vi "_Data Manager.vi"(5 "Error IN":errorcluster, 8 "Action":T1) -> (14 "Table":string[][](table), 19 "Error OUT":errorcluster)   [LabVIEW 2011]
uses:
  Controls/Data Manager Action.ctl
  Driver/Serial RS485/Controls/Serial_Action_Enum.ctl
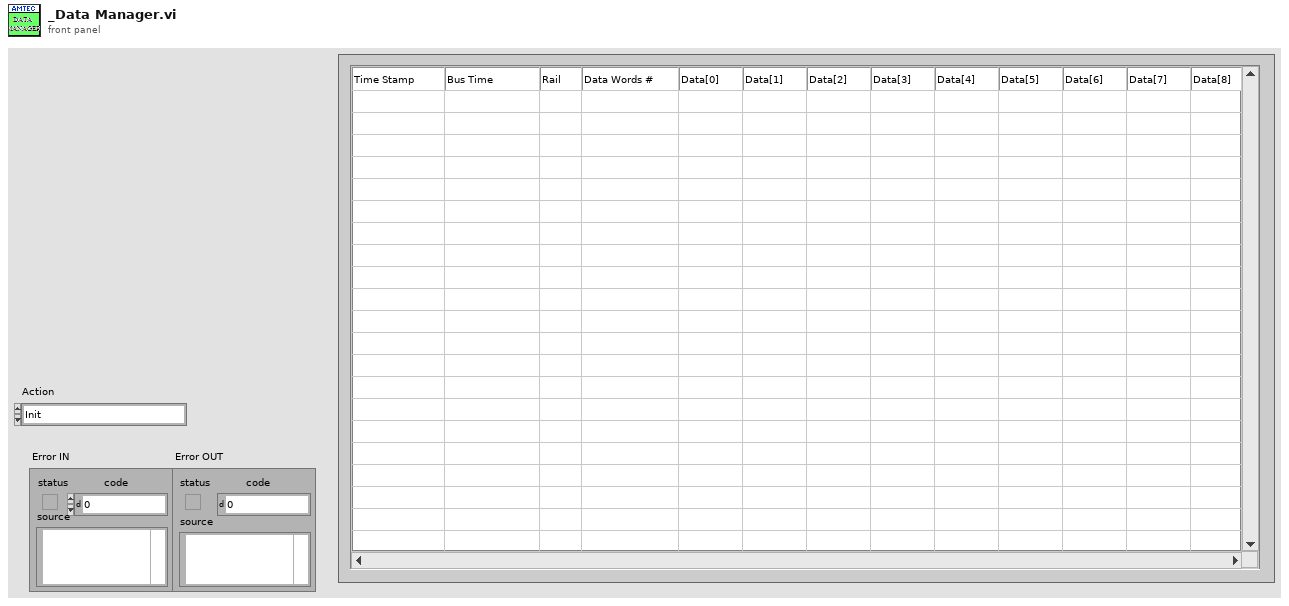
[diagram p1: front panel]
types:
  T1 = typedef "Data Manager Action.ctl" = enum16{"Init", "Status", "Get Data", "Get Log File Path", "Write Header", "Log Data", "Clear Table Data"}
  T2 = typedef "Serial_Action_Enum.ctl" = enum16{"Init", "Status", "Close", "Read All Chan", "Set Read Start Bit", "Clear Read Start Bit", "Read Beat", "Set RS485 Settings", "Close Ref"}
  T3 = typedef "Serial Data Cluster.ctl" = cluster{"String_Chan_1":string, "String_Chan_2":string, "String_Chan_3":string, "String_Chan_4":string, "#of Element Read Chan _1":i32, "#of Element Read Chan _2":i32, "#of Element Read Chan _3":i32, "#of Element Read Chan _4":i32, "Chan_1":timestamp, "Chan_2":timestamp, "Chan_3":timestamp, "Chan_4":timestamp}
  T4 = cluster{"Main Panel Path":path, "Config Directory":path, "Log Directory":path}
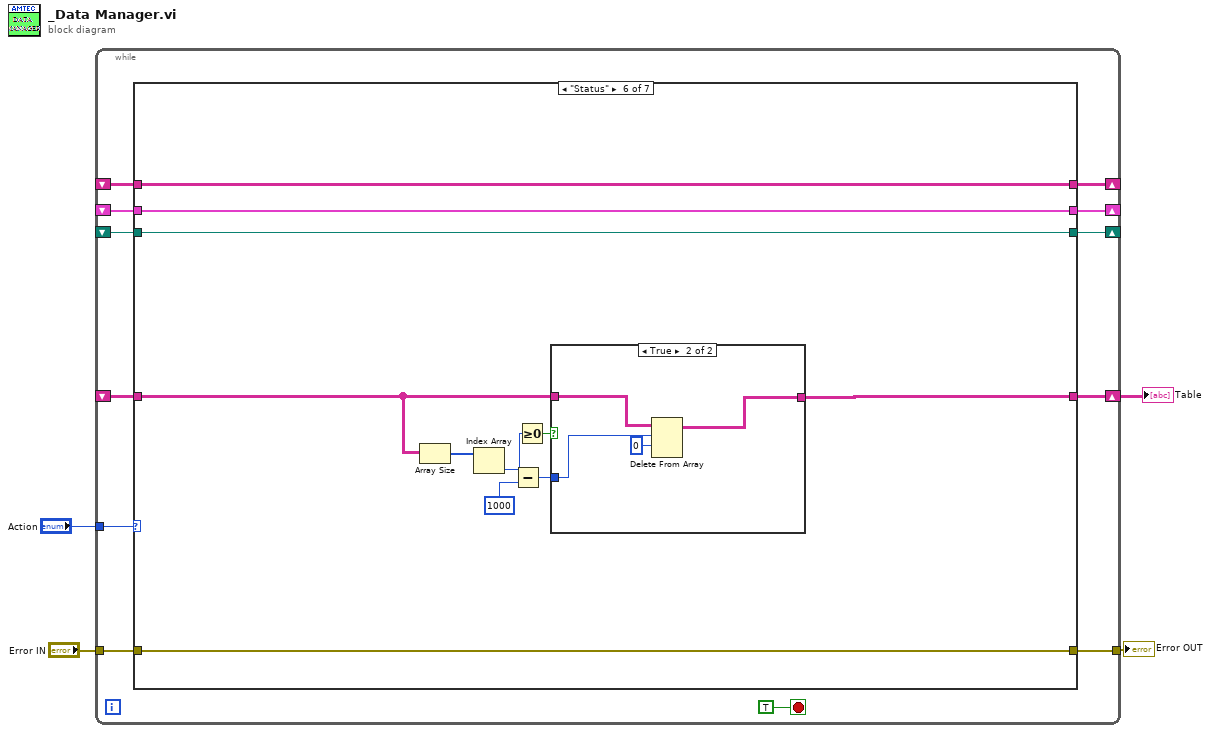
[diagram p0: block diagram]
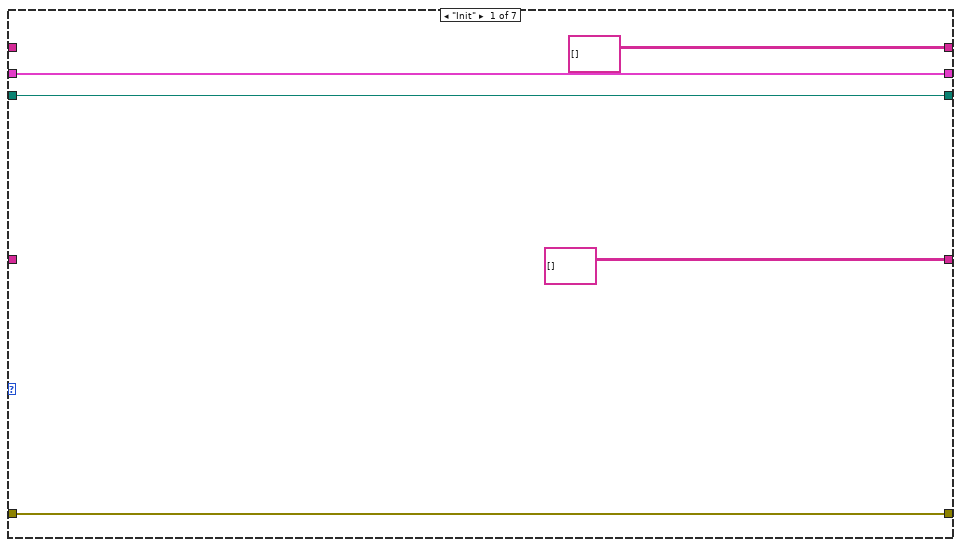
[diagram p2: hidden frame]
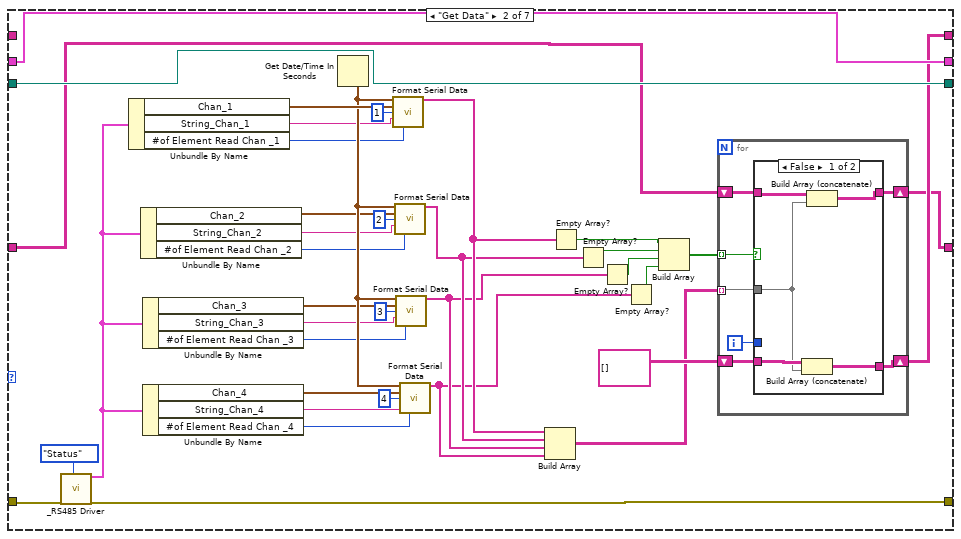
[diagram p3: hidden frame]
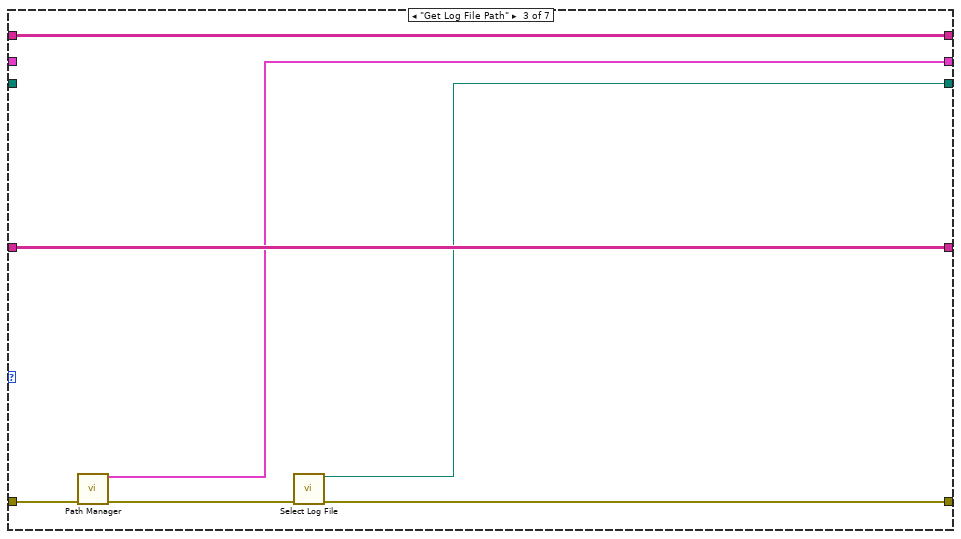
[diagram p5: hidden frame]
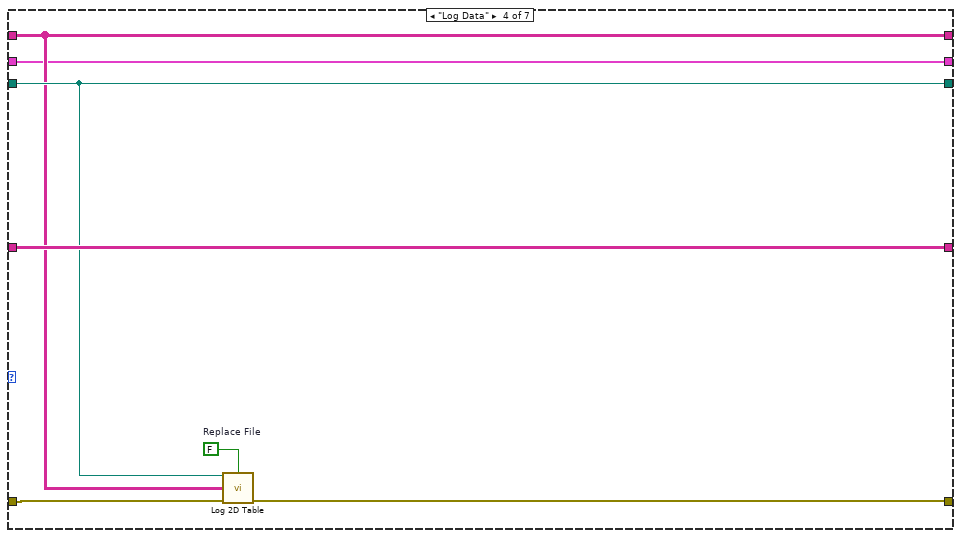
[diagram p6: hidden frame]
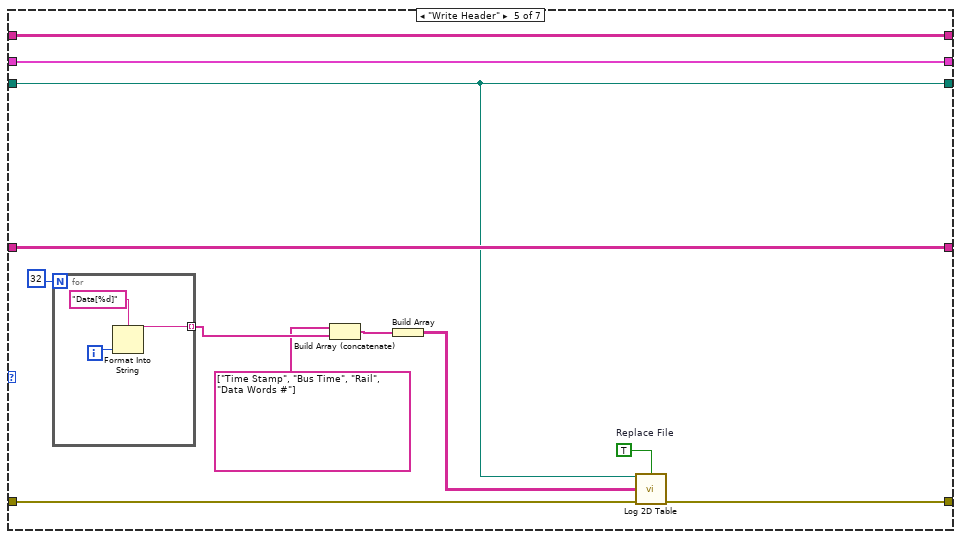
[diagram p7: hidden frame]
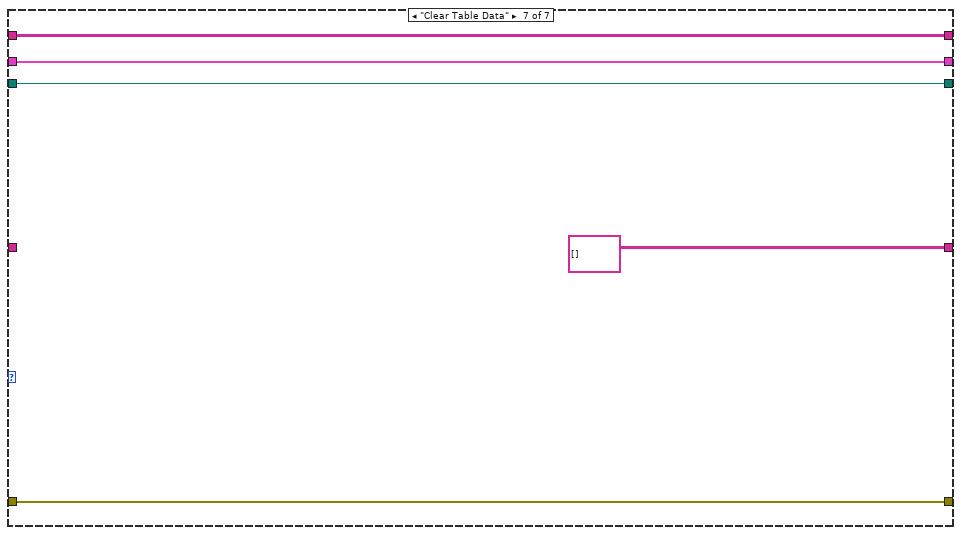
[diagram p9: hidden frame]
diagram:
  n1 = while {
    tunnel: "Action" -> [w15]
    tunnel: "Error IN" -> [w14]
    tunnel: [w13] -> w3
    shift-right: [w12] -> w1
    shift-left: _ -> [w11]
    shift-right: [w10] -> _
    shift-left: _ -> [w9]
    shift-right: [w8] -> _
    shift-left: _ -> [w7]
    shift-right: [w6] -> _
    shift-left: _ -> [w5]
    stop <- TRUE stop-if-true
    n2 = case shown="\"Status\"" w15 {
      tunnel: w14 -> [w21 w58 w77 w85 w93 w112 w122]
      tunnel: [w21 w57 w73 w82 w91 w112 w122] -> w13
      tunnel: [string[][] [] ("Results Table") w22 w79 w86 w98 w104 string[][] [] ("Results Table")] -> w12
      tunnel: w11 -> [_ w31 w79 w86 w98 w105 _]
      tunnel: [string[][] [] w23 w78 w83 w97 w111 w121] -> w10
      tunnel: w9 -> [_ _ w78 w83 w97 w111 w121]
      tunnel: [w18 w37 w76 w81 w88 w110 w120] -> w8
      tunnel: w7 -> [w18 w37 _ w81 w88 w110 w120]
      tunnel: [w17 w36 w74 w84 w92 w109 w119] -> w6
      tunnel: w5 -> [w17 w36 _ w84 w92 w109 w119]
      frame "Init" {
      }
      frame "Get Data" {
        n3 = call "_RS485 Driver.vi"("Error IN"=w58, "Action"=Serial_Action_Enum."Status") -> ("Serial Data Out"=w46:T3, "Error OUT"=w57:errorcluster)  [unwired: 15 in, 1 out]
        n4 = Unbundle By Name(w46) -> ("Chan_1"=w55:timestamp, "String_Chan_1"=w38:string, "#of Element Read Chan _1"=w45:i32)
        n5 = Unbundle By Name(w46) -> ("Chan_2"=w51:timestamp, "String_Chan_2"=w39:string, "#of Element Read Chan _2"=w44:i32)
        n6 = Unbundle By Name(w46) -> ("Chan_3"=w52:timestamp, "String_Chan_3"=w40:string, "#of Element Read Chan _3"=w43:i32)
        n7 = Unbundle By Name(w46) -> ("Chan_4"=w53:timestamp, "String_Chan_4"=w41:string, "#of Element Read Chan _4"=w42:i32)
        n8 = Get Date/Time In Seconds() -> (seconds since 1Jan1904=w54:timestamp)
        n9 = call "Format Serial Data.vi"("Time Stamp"=w54, "Bus Time"=w55, "Rail"=1, "String"=w38, "#of Element Read"=w45) -> ("Formatted Data"=w29:string[])  [unwired: 9 in, 1 out]
        n10 = call "Format Serial Data.vi"("Time Stamp"=w54, "Bus Time"=w51, "Rail"=2, "String"=w39, "#of Element Read"=w44) -> ("Formatted Data"=w28:string[])  [unwired: 9 in, 1 out]
        n11 = call "Format Serial Data.vi"("Time Stamp"=w54, "Bus Time"=w52, "Rail"=3, "String"=w40, "#of Element Read"=w43) -> ("Formatted Data"=w27:string[])  [unwired: 9 in, 1 out]
        n12 = call "Format Serial Data.vi"("Time Stamp"=w54, "Bus Time"=w53, "Rail"=4, "String"=w41, "#of Element Read"=w42) -> ("Formatted Data"=w26:string[])  [unwired: 9 in, 1 out]
        n13 = Build Array(w29, w28, w27, w26) -> (w24:string[][])
        n14 = Empty Array?(array=w29) -> (empty?=w35:bool)
        n15 = Empty Array?(array=w28) -> (empty?=w34:bool)
        n16 = Empty Array?(array=w27) -> (empty?=w33:bool)
        n17 = Empty Array?(array=w26) -> (empty?=w32:bool)
        n18 = Build Array(w35, w34, w33, w32) -> (w30:bool[])
        n19 = for {
          shift-right: [w63] -> w22
          shift-left: w31 -> [w64]
          tunnel: w30 -> [w65] mode=indexing
          tunnel: w24 -> [w62] mode=indexing
          shift-right: [w59] -> w23
          shift-left: string[][] [] ("appended array") -> [w60]
          i -> [w61]
          n20 = case shown="False" w65 {
            tunnel: [w70 w72] -> w63
            tunnel: w64 -> [w69 w72]
            tunnel: w62 -> [w66 _]
            tunnel: w61 -> [_ _]
            tunnel: w60 -> [w68 w71]
            tunnel: [w67 w71] -> w59
            frame False {
              n21 = Build Array (concatenate)(w68, w66) -> (w67:string[][])
              n22 = Build Array (concatenate)(w69, w66) -> (w70:string[][])
            }
            frame True {
            }
          }
        }
      }
      frame "Get Log File Path" {
        n23 = call "Path Manager.vi"("Error IN"=w77) -> ("Path Location Cluster"=w76:T4, "Error OUT"=w75:errorcluster)  [unwired: 13 in]
        n24 = call "Select Log File.vi"("Error IN"=w75) -> ("Log File OUT"=w74:path, "Error OUT"=w73:errorcluster)  [unwired: 13 in]
      }
      frame "Log Data" {
        w80 = FALSE  # Replace File
        n25 = call "Log 2D Table.vi"("Log Path"=w84, "Replace File"=w80, "Table Data IN"=w83, "Error IN"=w85) -> ("Error OUT"=w82:errorcluster)  [unwired: 11 in]
      }
      frame "Write Header" {
        w87 = TRUE  # Replace File
        n26 = for {
          N: 32 -> [_]
          tunnel: [w99] -> w96 mode=indexing
          i -> [w101]
          n27 = Format Into String(format string="Data[%d]", w101) -> (resulting string=w99:string)  [unwired: 2 in, 1 out]
        }
        n28 = Build Array (concatenate)(string[] ["Time Stamp", "Bus Time", "Rail", "Data Words #"] ("Column Header Strings[]"), w96) -> (w90:string[])
        n29 = Build Array(w90) -> (w89:string[][])
        n30 = call "Log 2D Table.vi"("Log Path"=w92, "Replace File"=w87, "Table Data IN"=w89, "Error IN"=w93) -> ("Error OUT"=w91:errorcluster)  [unwired: 11 in]
      }
      frame "Status" {
        n31 = Array Size(array=w105) -> (size(s)=w108:i32[])
        n32 = Index Array(array=w108) -> (element=w106:i32)  [unwired: 1 in]
        n33 = Subtract(x=w106, y=1000) -> (x-y=w103:i32)
        n34 = Greater Or Equal To 0?(x=w103) -> (x >= 0?=w102:bool)
        n35 = case shown="True" w102 {
          tunnel: w105 -> [w113 w117]
          tunnel: w103 -> [_ w115]
          tunnel: [w113 w114] -> w104
          frame False {
          }
          frame True {
            n36 = Delete From Array(array=w117, length=w115, index (row)=0) -> (array with subset deleted=w114:string[][])  [unwired: 1 in, 1 out]
          }
        }
      }
      frame "Clear Table Data" {
      }
    }
  }
  "Error OUT" <- w3
  "Table" <- w1
